vi "readRequest.vi"(5 "id":u16, 7 "cmd":string) -> (8 "readRequest":string)   [LabVIEW 2015]
panel:
  out "输出":u8[](array[numeric]) format="%02d"
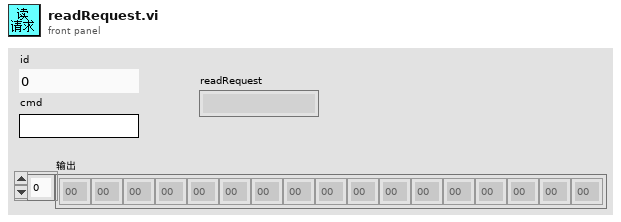
[diagram p1: front panel]
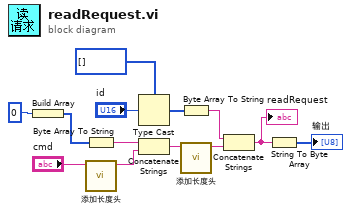
[diagram p0: block diagram]
diagram:
  n1 = Build Array(u8 0) -> (w7:u8[])
  n2 = Byte Array To String(unsigned byte array=w7) -> (string=w10:string)
  n3 = call "添加长度头.vi"("cmd"="cmd") -> ("添加后"=w11:string)  [unwired: 10 in]
  n4 = Type Cast(type=u8[] [], x="id") -> (*(type *) &x=w1:u8[])
  n5 = Concatenate Strings(w10, w11) -> (w9:string)
  n6 = Byte Array To String(unsigned byte array=w1) -> (string=w4:string)
  n7 = call "添加长度头.vi"("cmd"=w9) -> ("添加后"=w6:string)  [unwired: 10 in]
  n8 = Concatenate Strings(w4, w6) -> (w5:string)
  "readRequest" <- w5
  n9 = String To Byte Array(string=w5) -> (unsigned byte array=→"输出":u8[])
